vi "Select_Bookmark.vi"(8 "error in (no error)":errorcluster, 9 "Bookmark String":string, 11 "Documents Refnum in":refnum<k7>) -> (0 "error out":errorcluster, 3 "Documents Refnum Out":refnum<k7>)   [LabVIEW 2014]
panel:
  out "Selected Bookmark's Reference":refnum<k7>
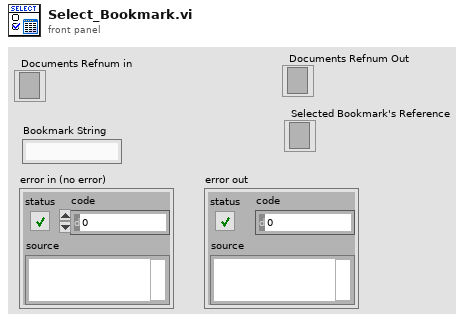
[diagram p1: front panel]
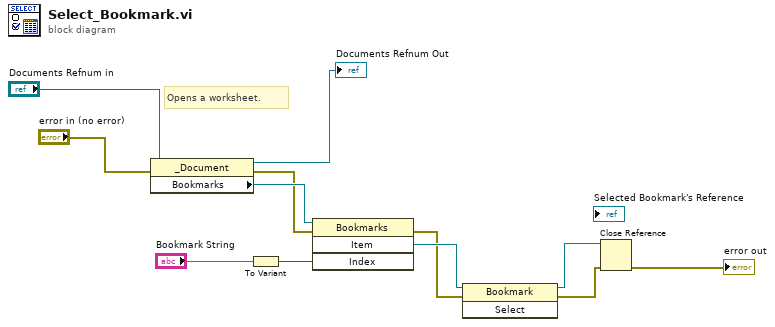
[diagram p0: block diagram]
diagram:
  # "Opens a worksheet."
  n1 = property class="_Document"(reference="Documents Refnum in", error in="error in (no error)") -> (reference out=→"Documents Refnum Out":refnum<k7>, error out=w6:errorcluster, "Bookmarks"=w9:refnum<k7>)
  n2 = To Variant(anything="Bookmark String") -> (Variant=w8:variant)
  n3 = invoke class="Bookmarks" method="Item"(reference=w9, error in=w6, "Index"=w8) -> (error out=w4:errorcluster, "Item"=w5:refnum<k7>)  [unwired: 1 in, 2 out]
  n4 = invoke class="Bookmark" method="Select"(reference=w5, error in=w4) -> (reference out=w3:refnum<k7>, error out=w2:errorcluster)  [unwired: 1 in, 1 out]
  n5 = Close Reference(reference=w3, error in (no error)=w2) -> (error out=→"error out":errorcluster)
